vi "Resistivity Calculate P.vi"(6 "Current Level (A)":dbl=0.1 min=5e-13 max=0.1 format="%#_6f", 7 "V1-V8 VDP":dbl[](array[numeric]), 8 "error in (no error)":errorcluster, 9 "fB":dbl=1.0 min=0.4 max=1.0, 10 "fA":dbl=1.0 min=0.4 max=1.0, 11 "Thickness (cm)":dbl) -> (0 "error out":errorcluster, 1 "pB":dbl, 2 "pA":dbl, 3 "pAVG":dbl)   [LabVIEW 2016, in "Hall Effect Library.lvlib"]
uses:
  Hall Effect Library.lvlib
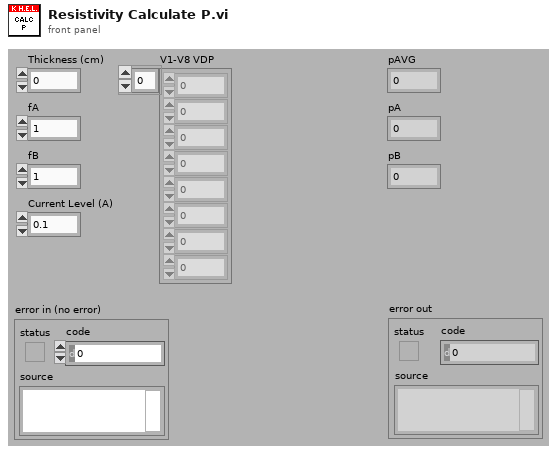
[diagram p1: front panel]
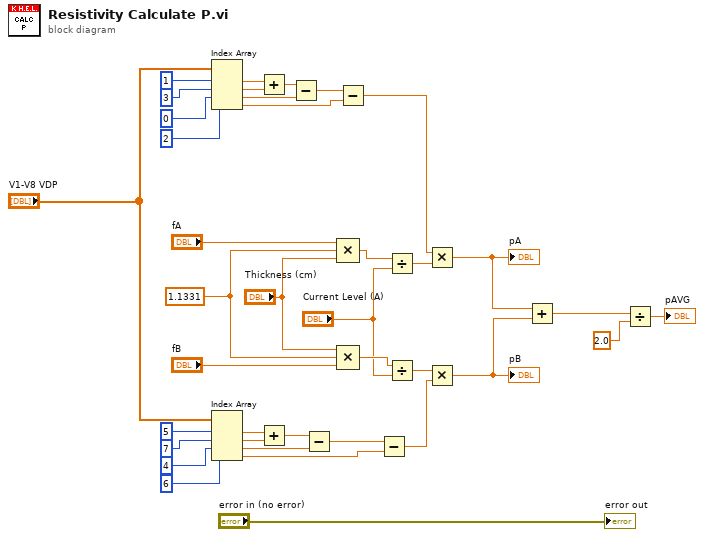
[diagram p0: block diagram]
diagram:
  w13 = 1.1331 ("pA")
  n1 = Index Array(array="V1-V8 VDP", index #1=1 ("index"), index #2=3 ("index"), index #3=0 ("index"), index #4=2 ("index")) -> (element #1=w12:dbl, element #2=w11:dbl, element #3=w9:dbl, element #4=w7:dbl)
  n2 = Index Array(array="V1-V8 VDP", index #1=5 ("index"), index #2=7 ("index"), index #3=4 ("index"), index #4=6 ("index")) -> (element #1=w6:dbl, element #2=w5:dbl, element #3=w3:dbl, element #4=w2:dbl)
  n3 = Add(x=w12, y=w11) -> (x+y=w10:dbl)
  n4 = Add(x=w6, y=w5) -> (x+y=w4:dbl)
  n5 = Subtract(x=w10, y=w9) -> (x-y=w8:dbl)
  n6 = Subtract(x=w4, y=w3) -> (x-y=w1:dbl)
  n7 = Compound Arithmetic op=MULTIPLY("fA", w13, "Thickness (cm)") -> (w26:dbl)
  n8 = Compound Arithmetic op=MULTIPLY("Thickness (cm)", w13, "fB") -> (w20:dbl)
  n9 = Subtract(x=w8, y=w7) -> (x-y=w24:dbl)
  n10 = Subtract(x=w1, y=w2) -> (x-y=w21:dbl)
  n11 = Divide(x=w26, y="Current Level (A)") -> (x/y=w25:dbl)
  n12 = Divide(x=w20, y="Current Level (A)") -> (x/y=w18:dbl)
  n13 = Multiply(x=w24, y=w25) -> (x*y=w17:dbl)
  "pA" <- w17
  n14 = Multiply(x=w18, y=w21) -> (x*y=w16:dbl)
  "pB" <- w16
  n15 = Add(x=w17, y=w16) -> (x+y=w15:dbl)
  n16 = Divide(x=w15, y=2.0) -> (x/y=→"pAVG":dbl)
  "error out" <- "error in (no error)"
